vi "AT Get String A.vi"(8 "error in (no error)":errorcluster, 10 "Feature":string, 11 "Handle":i32) -> (0 "error out":errorcluster, 2 "String":string, 3 "Status":i32)   [LabVIEW 2009]
doc: "Get String \n\nOutput:\n I32 Status\n String Value\n\nParameters:\n I32 Handle\n String Feature\n\nThis function will return the current value of the specified string feature. An error will be returned if the feature is currently not readable, not a string feature or is not implemented by the camera."
uses:
  atcoreA.dll
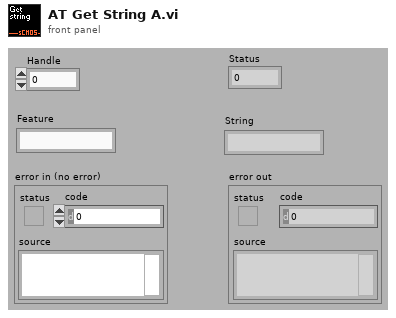
[diagram p1: front panel]
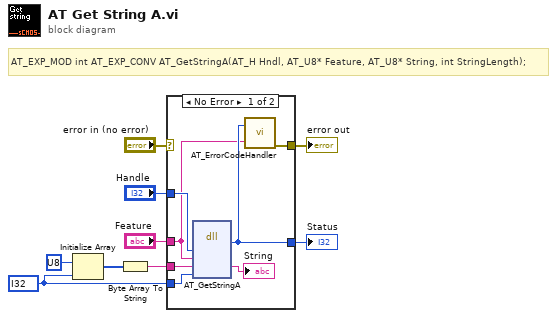
[diagram p0: block diagram]
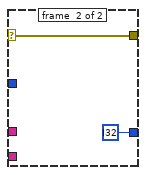
[diagram p2: hidden frame]
diagram:
  w3 = i32 ? ("dimension size")
  # "AT_EXP_MOD int AT_EXP_CONV AT_GetStringA(AT_H Hndl, AT_U8* Feature, AT_U8* String, int StringLength);"
  n1 = Initialize Array(u8 ? ("element"), w3) -> (w6:u8[])
  n2 = Byte Array To String(unsigned byte array=w6) -> (string=w4:string)
  n3 = case shown="No Error" "error in (no error)" {
    selector: "error in (no error)" -> [_ w18]
    tunnel: [w12 i32 ?] -> w9
    tunnel: "Handle" -> [w16 _]
    tunnel: "Feature" -> [w10 _]
    tunnel: w4 -> [w14 _]
    tunnel: w3 -> [w13 _]
    tunnel: [w11 w18] -> w2
    frame #0 {
      n4 = dll-call lib="atcoreA.dll" fn="AT_GetStringA"("Handle"=w16, "Feature"=w10, "String"=w14, "StringLength"=w13) -> ("Status"=w12:i32, "String"=→"String":string)  [unwired: 6 in, 2 out]
      n5 = call "AT_ErrorCodeHandler.vi"("Error"=w12, "Feature Name"=w10) -> ("error out"=w11:errorcluster)  [unwired: 5 in]
    }
    frame #1 {
    }
  }
  "Status" <- w9
  "error out" <- w2
